vi "Swerve_Module Azimuth Config.vi"(5 "Max # Of Tries":i32=3, 6 "Send Cmd Timout(ms)":u32=300, 7 "Specific Data":T1, 8 "Error":errorcluster, 9 "Module Azimuth Config Data":T8={"ModuleAzimuth Ver"=0, "Output"={"Type"=enum."Counter-Clockwise", "Neutral"=enum."EEPROMSetting", "Max"={"FWD"=0.0, "REV"=0.0}, "Min"={"FWD"=0.04, "REV"=0.0}, "OL Ramp Rate (S)"=0.0, "Dead Band"=0.0}, "CL"={"Gains"={"P"=1.0, "I"=0.01, "D"=0.0, "F"=0.0}, "Error Allowed"={"High"=0.0, "Low"=0.0}, "I Zone"={"High"=10000.0, "Low"=-1000.0}, "Max Out"={"FWD"=1.0, "REV"=-1.0}, "Max I Accu"={"High"=10.0, "Low"=-10.0}, "CL Ramp Rate (S)"=0.0}, "MM"={"Cruise Velocity"=5000, "Acceleration"=5000}} {"Output"."Min"."REV" format="%.2f"; "Output"."Min"."FWD" format="%.2f"; "Output"."Max"."REV" format="%.2f"; "Output"."Max"."FWD" format="%.2f"; "CL"."Max I Accu"."Low" format="%#.8f"; "CL"."Max I Accu"."High" format="%#.8f"; "CL"."Gains"."F" format="%#.8f"; "CL"."Gains"."D" format="%#.8f"; "CL"."Gains"."I" format="%#.8f"; "CL"."Gains"."P" format="%#.8f"; "CL"."Error Allowed"."Low" format="%#.8f"; "CL"."Error Allowed"."High" format="%#.8f"; "CL"."I Zone"."Low" format="%#.8f"; "CL"."I Zone"."High" format="%#.8f"; "CL"."Max Out"."REV" format="%.2f"; "CL"."Max Out"."FWD" format="%.2f"}, 11 "PhoenixMotorControlDevRef":T3={"DeviceStatus"={"status"=FALSE, "code"=0, "source"=""}, "Type"=enum."PWM", "PWM"={"PWM Channel"=enum."Invalid", "DeadBand"={"Name"="", "maxPositivePwm"=0, "minPositivePwm"=0, "centerPwm"=0, "maxNegativePwm"=0, "minNegativePwm"=0, "angularRange"=0}}, "CAN"={"Device Number"=0, "SetOutput VI Ref"=variant, "GetOutput VI Ref"=variant, "Enable VI Ref"=variant, "Disable VI Ref"=variant, "Data"=variant}, "Invert"=FALSE, "DIO PWM"={"PWM \"Enable\" Channel"=enum."Invalid", "DIOChannel"=enum."Invalid", "PWM Rate"=0.0}}) -> (0 "Error Out":errorcluster, 3 "Module Azimuth Ref Out":T3)   [LabVIEW 2023]
uses:
  <vilib>/Utility/Data Type/NI_Data Type.lvlib
  <vilib>/Rock Robotics/WPI/ThirdParty/Phoenix-LabVIEW/Motor Controller/Controls/CTRE_Phoenix_MotorControl_RemoteSourceType.ctl
  <vilib>/Rock Robotics/WPI/ThirdParty/Phoenix-LabVIEW/Motor Controller/Controls/CTRE_Phoenix_MotorControl_FeedbackDevice_TalonFX.ctl
  <vilib>/Rock Robotics/SystemInterfaces/DIO/FPGA_DIOPWMChannel.ctl
  <vilib>/Rock Robotics/WPI/PWM/WPI_PWMDeadband.ctl
  <vilib>/Rock Robotics/WPI/MotorControl/WPI_MotorControlType.ctl
  <vilib>/Rock Robotics/SystemInterfaces/DIO/FPGA_DIOChannel.ctl
  <vilib>/Rock Robotics/WPI/MotorControl/WPI_MotorControlDeviceRef.ctl
  Shared Code/TypeDefs/Cluster_Motion Magic Parameters.ctl
  Shared Code/TypeDefs/Cluster_High-Low.ctl
  Shared Code/TypeDefs/Cluster_PID Gains.ctl
  Shared Code/TypeDefs/Cluster_PID Config.ctl
  <vilib>/Rock Robotics/WPI/ThirdParty/Phoenix-LabVIEW/Motor Controller/Controls/CTRE_Phoenix_MotorControl_TalonFXInvertType.ctl
  <vilib>/Rock Robotics/WPI/ThirdParty/Phoenix-LabVIEW/Motor Controller/Controls/CTRE_Phoenix_MotorControl_NeutralMode.ctl
  Shared Code/TypeDefs/Cluster_Swerve Module Azimuth Config Data.ctl
  Shared Code/TypeDefs/ENUM_Motor Index.ctl
  Shared Code/TypeDefs/Cluster_Module Specific Config Data.ctl
  Shared Code/TypeDefs/Cluster_FWD  REV Values.ctl
  Shared Code/TypeDefs/Cluster_Config Motor Output.ctl
panel:
  # "Tune Output\nto 1023 Max"
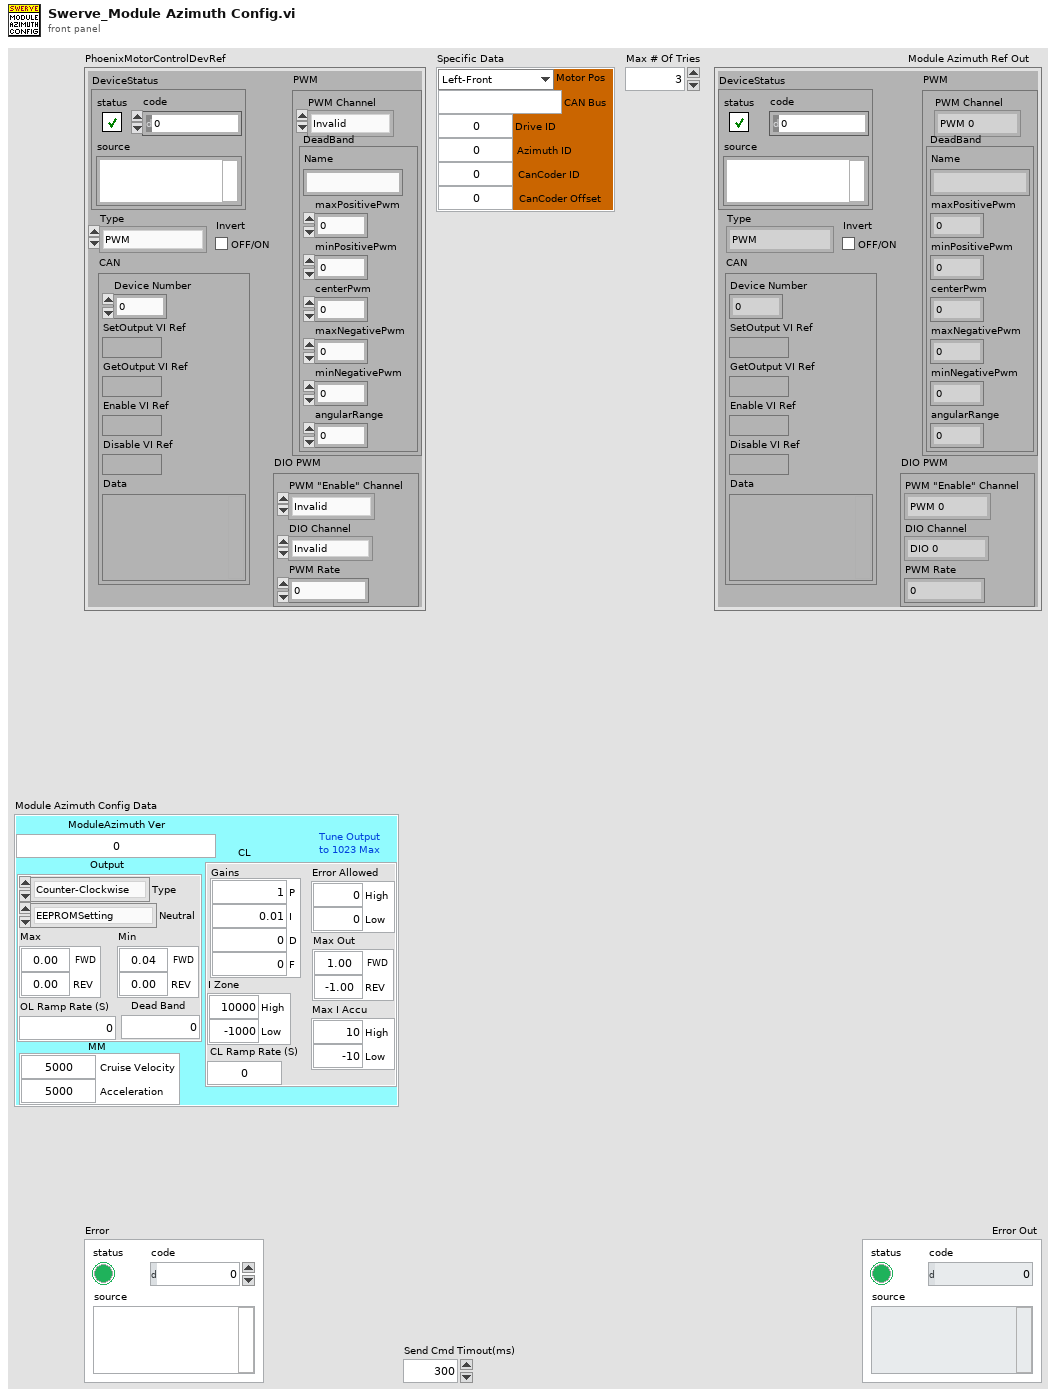
[diagram p1: front panel]
types:
  T1 = typedef "Cluster_Module Specific Config Data.ctl" = cluster{"Motor Pos":T2, "CAN Bus":string, "Drive ID":u8, "Azimuth ID":u8, "CanCoder ID":u8, "CanCoder Offset":dbl}
  T2 = typedef "ENUM_Motor Index.ctl" = enum16{"Left-Front", "Right-Front", "Left-Back", "Right-Back"}
  T3 = typedef "WPI_MotorControlDeviceRef.ctl" = cluster{"DeviceStatus":errorcluster, "Type":T4, "PWM":cluster{"PWM Channel":T5, "DeadBand":T6}, "CAN":cluster{"Device Number":u8, "SetOutput VI Ref":variant, "GetOutput VI Ref":variant, "Enable VI Ref":variant, "Disable VI Ref":variant, "Data":variant}, "Invert":bool, "DIO PWM":cluster{"PWM \"Enable\" Channel":T5, "DIOChannel":T7, "PWM Rate":dbl}}
  T4 = typedef "WPI_MotorControlType.ctl" = enum16{"PWM", "CAN", "DIO PWM"}
  T5 = typedef "FPGA_DIOPWMChannel.ctl" = enum8{"PWM 0", "PWM 1", "PWM 2", "PWM 3", "PWM 4", "PWM 5", "PWM 6", "PWM 7", "PWM 8", "PWM 9", "PWM MXP 0", "PWM MXP 1", "PWM MXP 2", "PWM MXP 3", "PWM MXP 4", "PWM MXP 5", "PWM MXP 6", "PWM MXP 7", "PWM MXP 8", "PWM MXP 9", "Invalid"}
  T6 = typedef "WPI_PWMDeadband.ctl" = cluster{"Name":string, "maxPositivePwm":i32, "minPositivePwm":i32, "centerPwm":i32, "maxNegativePwm":i32, "minNegativePwm":i32, "angularRange":u16}
  T7 = typedef "FPGA_DIOChannel.ctl" = enum8{"DIO 0", "DIO 1", "DIO 2", "DIO 3", "DIO 4", "DIO 5", "DIO 6", "DIO 7", "DIO 8", "DIO 9", "DIO MXP 0", "DIO MXP 1", "DIO MXP 2", "DIO MXP 3", "DIO MXP 4", "DIO MXP 5", "DIO MXP 6", "DIO MXP 7", "DIO MXP 8", "DIO MXP 9", "DIO MXP 10", "DIO MXP 11", "DIO MXP 12", "DIO MXP 13", "DIO MXP 14", "DIO MXP 15", "SPI Port CS1", "SPI Port CS2", "SPI Port CS3", "SPI Port MISO", "SPI Port MOSI", "Invalid"}
  T8 = typedef "Cluster_Swerve Module Azimuth Config Data.ctl" = cluster{"ModuleAzimuth Ver":u64, "Output":T9, "CL":T13, "MM":T16}
  T9 = typedef "Cluster_Config Motor Output.ctl" = cluster{"Type":T10, "Neutral":T11, "Max":T12, "Min":T12, "OL Ramp Rate (S)":dbl, "Dead Band":dbl}
  T10 = typedef "CTRE_Phoenix_MotorControl_TalonFXInvertType.ctl" = enum16{"Counter-Clockwise", "Clockwise"}
  T11 = typedef "CTRE_Phoenix_MotorControl_NeutralMode.ctl" = enum8{"EEPROMSetting", "Override to Coast", "Override to Brake"}
  T12 = typedef "Cluster_FWD  REV Values.ctl" = cluster{"FWD":dbl, "REV":dbl}
  T13 = typedef "Cluster_PID Config.ctl" = cluster{"Gains":T14, "Error Allowed":T15, "I Zone":T15, "Max Out":T12, "Max I Accu":T15, "CL Ramp Rate (S)":dbl}
  T14 = typedef "Cluster_PID Gains.ctl" = cluster{"P":dbl, "I":dbl, "D":dbl, "F":dbl}
  T15 = typedef "Cluster_High-Low.ctl" = cluster{"High":dbl, "Low":dbl}
  T16 = typedef "Cluster_Motion Magic Parameters.ctl" = cluster{"Cruise Velocity":i32, "Acceleration":i32}
  T17 = typedef "CTRE_Phoenix_MotorControl_RemoteSourceType.ctl" = enum16{"Off", "Talon SRX Selected Sensor", "Pigeon IMU Yaw", "Pigeon IMU Pitch", "Pigeon IMU Roll", "CANifier Quadrature", "CANifier PWM Input 0", "CANifier PWM Input 1", "CANifier PWM Input 2", "CANifier PWM Input 3", "Gadgeteer Pigeon Yaw", "Gadgeteer Pigeon Pitch", "Gadgeteer Pigeon Roll", "CANCoder"}
  T18 = typedef "CTRE_Phoenix_MotorControl_FeedbackDevice_TalonFX.ctl" = i8
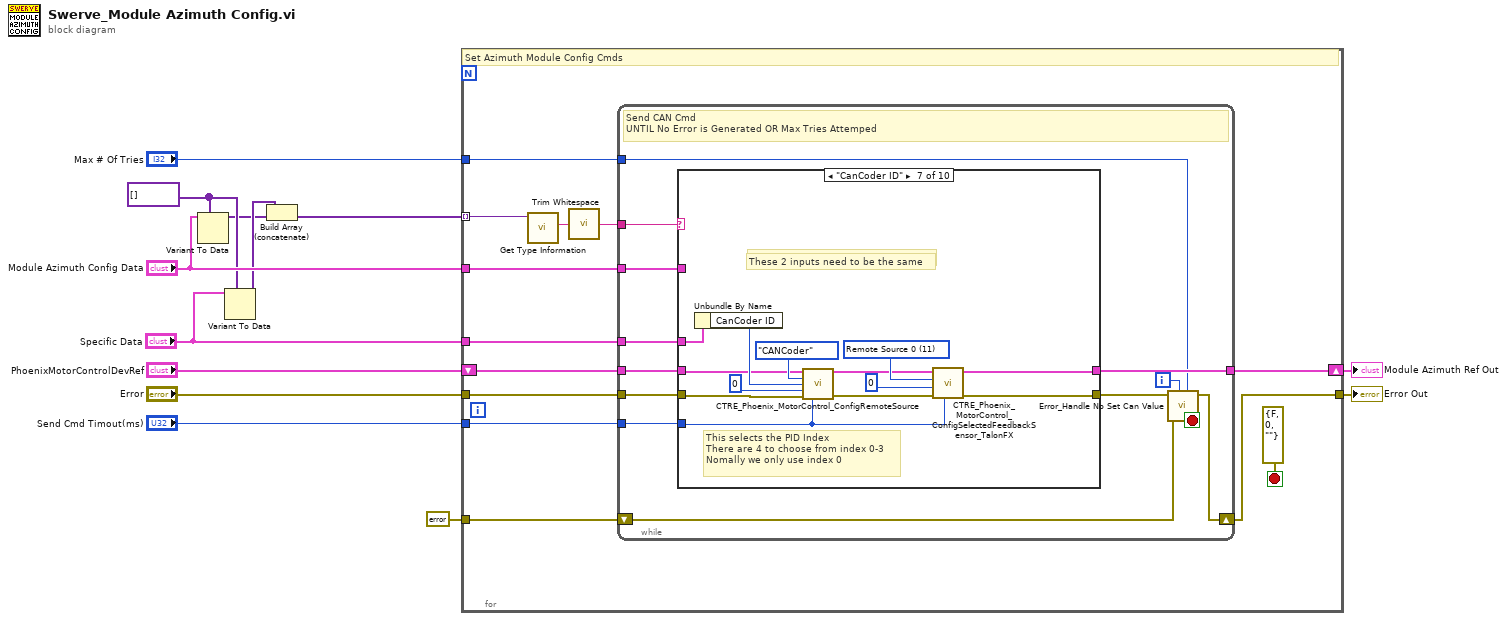
[diagram p0: block diagram]
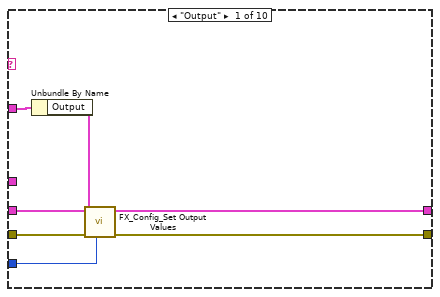
[diagram p2: hidden frame]
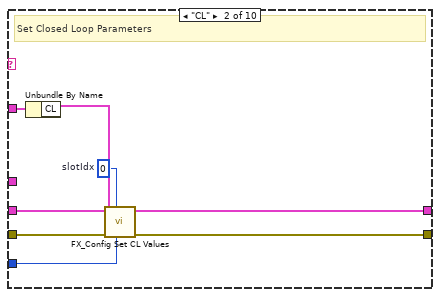
[diagram p3: hidden frame]
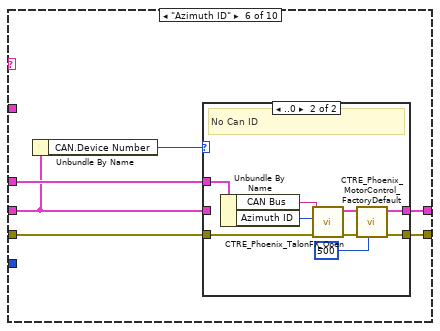
[diagram p7: hidden frame]
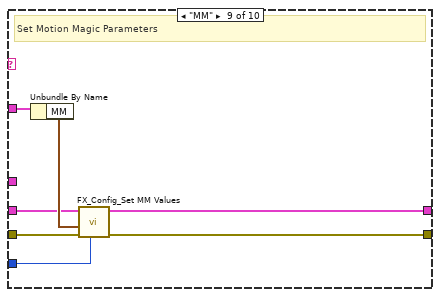
[diagram p10: hidden frame]
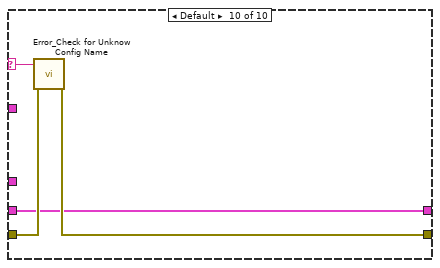
[diagram p11: hidden frame]
diagram:
  w4 = variant[] [] ("type")
  n1 = Variant To Data(type=w4, Variant="Module Azimuth Config Data") -> (data=w2:variant[])  [unwired: 1 in, 1 out]
  n2 = Variant To Data(type=w4, Variant="Specific Data") -> (data=w3:variant[])  [unwired: 1 in, 1 out]
  n3 = Build Array (concatenate)(w3, w2) -> (w1:variant[])
  n4 = for {
    tunnel: "Send Cmd Timout(ms)" -> [w25]
    tunnel: errorcluster {"status"=FALSE, "code"=0, "source"=""} ("Error Out") -> [w23]
    shift-right: [w26] -> w13
    shift-left: "PhoenixMotorControlDevRef" -> [w22]
    tunnel: "Module Azimuth Config Data" -> [w24]
    tunnel: "Max # Of Tries" -> [w20]
    tunnel: w1 -> [w19] mode=indexing
    tunnel: "Error" -> [w21]
    tunnel: [w18] -> w12
    tunnel: "Specific Data" -> [w16]
    stop <- errorcluster {"status"=FALSE, "code"=0, "source"=""} ("error IO") stop-if-true
    # "Set Azimuth Module Config Cmds"
    n5 = call <vilib>:"Get Type Information.vi"("variant"=w19) -> ("name"=w15:string)  [unwired: 6 in, 4 out]
    n6 = call <vilib>:"Trim Whitespace.vi"("string"=w15) -> ("trimmed string"=w14:string)  [unwired: 1 in]
    n7 = while {
      tunnel: [w32] -> w26
      tunnel: w25 -> [w37]
      shift-right: [w38] -> w18
      shift-left: w23 -> [w36]
      tunnel: w21 -> [w34]
      tunnel: w22 -> [w33]
      tunnel: w24 -> [w27]
      tunnel: w20 -> [w31]
      tunnel: w14 -> [w30]
      tunnel: w16 -> [w28]
      i -> [w35]
      stop <- w29 stop-if-true
      # "Send CAN Cmd\nUNTIL No Error is Generated OR Max Tries Attemped"
      n8 = case shown="\"CanCoder ID\"" w30 {
        selector: w30 -> [_ _ _ _ _ _ _ _ _ w100]
        tunnel: [w43 w53 w55 w57 w59 w63 w79 w92 w98 w102] -> w39
        tunnel: w37 -> [w40 w47 _ _ _ _ w81 _ w93 _]
        tunnel: w34 -> [w44 w54 w55 w57 w59 w64 w82 w92 w97 w103]
        tunnel: w33 -> [w42 w50 w56 w58 w60 w61 w83 w91 w94 w101]
        tunnel: [w45 w52 w56 w58 w60 w66 w80 w91 w99 w101] -> w32
        tunnel: w28 -> [_ _ _ _ _ w65 w78 _ _ _]
        tunnel: w27 -> [w46 w51 _ _ _ _ _ _ w96 _]
        frame "Output" {
          n9 = Unbundle By Name(w46) -> ("Output"=w41:T9)
          n10 = call "FX_Config_Set Output Values.vi"("Send Cmd Timout(ms)"=w40, "Error"=w44, "Output"=w41, "PhoenixMotorControlDevRef"=w42) -> ("Error Out"=w43:errorcluster, "PhoenixMotorControlDevRef Out"=w45:T3)  [unwired: 6 in]
        }
        frame "CL" {
          w48 = 0  # slotIdx
          # "Set Closed Loop Parameters"
          n11 = Unbundle By Name(w51) -> ("CL"=w49:T13)
          n12 = call "FX_Config Set CL Values.vi"("Send Cmd Timout(ms)"=w47, "SlotIdx"=w48, "Error"=w54, "CL"=w49, "PhoenixMotorControlDevRef"=w50) -> ("Error Out"=w53:errorcluster, "PhoenixMotorControlDevRef Out"=w52:T3)  [unwired: 4 in, 1 out]
        }
        frame "Motor Pos" {
        }
        frame "CAN Bus" {
        }
        frame "Drive ID" {
        }
        frame "Azimuth ID" {
          n13 = Unbundle By Name(w61) -> ("CAN.Device Number"=w62:u8)
          n14 = case shown="..0" w62 {
            tunnel: [w68 w73] -> w66
            tunnel: w65 -> [_ w72]
            tunnel: w64 -> [w67 w71]
            tunnel: [w67 w70] -> w63
            tunnel: w61 -> [w68 _]
            frame 1.. {
              # "CAN ID Already Open"
            }
            frame ..0 {
              # "No Can ID"
              n15 = Unbundle By Name(w72) -> ("CAN Bus"=w69:string, "Azimuth ID"=w74:u8)
              n16 = call <vilib>:"CTRE_Phoenix_TalonFX_Open.vi"("error in"=w71, "Device Number"=w74, "CAN Bus"=w69) -> ("error out"=w76:errorcluster, "PhoenixMotorControlDevRef"=w77:T3)  [unwired: 7 in]
              n17 = call <vilib>:"CTRE_Phoenix_MotorControl_FactoryDefault.vi"("timeoutMs"=500, "error in"=w76, "PhoenixMotorControlDevRef"=w77) -> ("error out"=w70:errorcluster, "PhoenixMotorControlDevRef"=w73:T3)  [unwired: 7 in]
            }
          }
        }
        frame "CanCoder ID" {
          w87 = T18 11 items=["Integrated Sensor"=1, "Sensor Sum (S0 + S1)"=9, "Sensor Difference (D0 - D1)"=10, "Remote Source 0"=11, "Remote Source 1"=12, "None"=14, "Software Emulated"=15] ("Talon FX Feedback Device")
          # "This selects the PID Index\nThere are 4 to choose from index 0-3\nNomally we only use index 0"
          # "These 2 inputs need to be the same"
          # "These 2 inputs need to be the same"
          n18 = Unbundle By Name(w78) -> ("CanCoder ID"=w88:u8)
          n19 = call <vilib>:"CTRE_Phoenix_MotorControl_ConfigRemoteSource.vi"("PhoenixMotorControlDevRef"=w83, "Remote Device Type"=CTRE_Phoenix_MotorControl_RemoteSourceType."CANCoder", "Remote Device ID"=w88, "Source Index (0/1)"=u32 0, "error in (no error)"=w82, "timeoutMs"=w81) -> ("PhoenixMotorControlDevRef"=w84:T3, "error out"=w85:errorcluster)  [unwired: 8 in]
          n20 = call <vilib>:"CTRE_Phoenix_MotorControl_ConfigSelectedFeedbackSensor_TalonFX.vi"("timeoutMs"=w81, "error in (no error)"=w85, "pidLoopIdx"=0, "Talon FX Feedback Device"=w87, "PhoenixMotorControlDevRef"=w84) -> ("error out"=w79:errorcluster, "PhoenixMotorControlDevRef"=w80:T3)  [unwired: 5 in]
        }
        frame "CanCoder Offset" {
        }
        frame "MM" {
          # "Set Motion Magic Parameters"
          n21 = Unbundle By Name(w96) -> ("MM"=w95:T16)
          n22 = call "FX_Config_Set MM Values.vi"("Send Cmd Timout(ms)"=w93, "Error"=w97, "MM"=w95, "PhoenixMotorControlDevRef"=w94) -> ("Error Out"=w98:errorcluster, "PhoenixMotorControlDevRef Out"=w99:T3)  [unwired: 6 in]
        }
        frame Default {
          n23 = call "Error_Check for Unknow Config Name.vi"("error in (no error)"=w103, "Config Name"=w100) -> ("error out"=w102:errorcluster)  [unwired: 9 in]
        }
      }
      n24 = call "Error_Handle No Set Can Value.vi"("Max # Of Tries"=w31, "Loop Itteration"=w35, "Previous Error"=w36, "Error"=w39) -> ("Stop Out"=w29:bool, "Error Out"=w38:errorcluster)  [unwired: 6 in]
    }
  }
  "Module Azimuth Ref Out" <- w13
  "Error Out" <- w12
